vi "report_test_27_5_A86b2.vi"() -> ()   [LabVIEW 2021]
uses:
  <vilib>/Utility/NIReport.llb/NI_report.lvclass
  <vilib>/Platform/TimedLoop/XDataNode/timing_clust.ctl
  <vilib>/Platform/TimedLoop/XDataNode/nitl_modes.ctl
  <vilib>/Platform/TimedLoop/XDataNode/wakeup.ctl
  <vilib>/Utility/NIReport.llb/Report Type.ctl
  <extravilib>/ChannelInstances/Tag-dbl/Read With Abort.vi
  <extravilib>/ChannelInstances/Tag-a[.](dbl)/Write With Abort.vi
  <extravilib>/ChannelInstances/Tag-bool/Write With Abort.vi
  <extravilib>/ChannelInstances/Tag-bool/Read With Abort.vi
  <extravilib>/ChannelInstances/Tag-a[.](dbl)/Read With Abort.vi
  <extravilib>/ChannelInstances/Tag-dbl/Write With Abort.vi
  <extravilib>/ChannelInstances/Tag-dbl/Instantiate.vi
  <extravilib>/ChannelInstances/Tag-bool/Instantiate.vi
  <extravilib>/ChannelInstances/Tag-bool/EndpointRead.vi
  <vilib>/OPCUA/client/Multiple Read Float.vi
  <extravilib>/ChannelInstances/Tag-dbl/Endpoint.vi
  <extravilib>/ChannelInstances/Tag-a[.](dbl)/Instantiate.vi
  <extravilib>/ChannelInstances/Tag-bool/Endpoint.vi
  <extravilib>/ChannelInstances/Tag-a[.](dbl)/EndpointRead.vi
  <vilib>/Utility/file.llb/Write Delimited Spreadsheet (DBL).vi
  <vilib>/Utility/NIReport.llb/Append Numeric Table to Report (wrap).vi
  <extravilib>/ChannelInstances/Tag-dbl/EndpointRead.vi
  <extravilib>/ChannelInstances/Tag-a[.](dbl)/Endpoint.vi
  <vilib>/Platform/TimedLoop/XDataNode/XDataNode.xnode
  <vilib>/Platform/TimedLoop/XDataNode/XDNodeRunTimeDep.lvlib
  <extravilib>/ChannelInstances/Tag-bool.lvlib
  <vilib>/OPCUA/NI OPC UA Client.lvlib
  <vilib>/Utility/NIReport.llb/NI_ReportGenerationCore.lvlib
  <extravilib>/ChannelInstances/Tag-a[.](dbl).lvlib
  <extravilib>/ChannelInstances/Tag-dbl.lvlib
panel:
  in  "y 2":dbl=1.5
  out "x":dbl
  out "highqq":dbl(graph)
  out "Endpoint_Highqq":dbl
  out "velx":dbl(graph)
  out "x":dbl(graph)
  out "vx":dbl
  out "angle Y":dbl
  out "Endpoint_l":dbl[](array[numeric])
  out "Endpoint_lfull 2":dbl[][](array[numeric])
  in  "source file path":path=path "D:/Phuc/postopulsem2.m"
  out "appended array 2":dbl[](array[numeric])
  out "appended array":dbl[](array[numeric])
  out "data out 2":string
  in  "String":string="Flight_report"
  out "Gyro acc & vel":dbl[](array[numeric])
  out "Roll & Pitch":cluster{"[0]":dbl, "[1]":dbl}(graph)
  out "Cable length":T1(graph)
  out "Tilt sensor array":dbl[](array[numeric])
  out "Cable length Array":dbl[](array[numeric])
  in  "PAR_GpDec":dbl=120000.0
  in  "Set pos":bool caption="Blank Button"
  in  "Set cmd & actual pos":dbl[](array[numeric])=[0.0, 0.0, 0.0, 0.0, 0.0, 0.0, -2293.0, -3672.0]
  in  "CFG_GpSFEnable":u32(ring) items=["SF_Disable", "SF_Enable"]
  in  "Par":bool
  out "Ax = y?":bool
  in  "CFG_GpBldTime":u32
  in  "y":u32=1
  out "pCurIndex":u32
  out "pCurCmdFunc":u32
  out "pRemainCount":u32
  out "pFreeSpaceCount":u32
  out "Waveform Chart":T1(graph)
  out "Tensile force array":dbl[](array[numeric])
  out "Exel report":refnum<class "NI_report.lvclass">
  out "Roll":string
  out "Pitch":string
  out "Yaw":string="0"
  out "LinAcc X":string
  out "LinAcc Y":string
  out "LinAcc Z":string
  out "Cable velocity (m/s)":T1(graph)
  in  "Tab Control":enum32{"Page 1", "Page 2"}(tab)
  in  "Open Board":bool
  in  "Stop 2":bool
  out "Group State:":string
  in  "Servo On":bool
  in  "Adress":string="192.168.0.100"
  in  "Port 2":u16=3535
  in  "bytes to read 2":i32=32
  in  "Stop 3":bool
  in  "bytes to read":i32=72
  in  "Address":string="192.168.0.199"
  in  "Port":u16=8888
  in  "stop":bool
  in  "Clear report":bool
  in  "Save report":bool
  in  "Enable write":bool
  in  "Write to report":bool
  in  "Close Board":bool
  in  "trust any server (F)":bool=TRUE
  in  "Server endpoint URL":string="opc.tcp://127.0.0.1:49350"
  in  "NodeID 8":string="ns=2;s=S7.PLC4.loadcell7"
  in  "NodeID 7":string="ns=2;s=S7.PLC4.loadcell6"
  in  "NodeID 6":string="ns=2;s=S7.PLC3.loadcell5"
  in  "NodeID 5":string="ns=2;s=S7.PLC3.loadcell4"
  in  "NodeID 3":string="ns=2;s=S7.PLC2.loadcell2"
  in  "NodeID 4":string="ns=2;s=S7.PLC2.loadcell3"
  in  "NodeID 2":string="ns=2;s=S7.PLC1.loadcell1"
  in  "NodeID 1":string="ns=2;s=S7.PLC1.loadcell0"
  out "data out":string
  out "Measured tensile force (N)":T2(graph)
  out "Error Code:":u32 format="%x"
  out "Error Msg":string
  out "Error":bool
  in  "Reset Error":bool
  out "Instrument":string="If you want to exit program,Please press \"Exit Program\" button"
  out "DeviceNum List":u32[](array[numeric])
  out "Servo_Off":bool
  out "Servo_On":bool
  out "GPHandle":u64
  out "CFG_GpAxesInGroup":u32
  out "GroupClosed":bool
  out "GroupStopped":bool
  out "DirectAbsSuccess":bool
  out "DirectRelSuccess":bool
  in  "Movement Mode":enum32{"Absolute", "Relative"}(radio)=enum."Relative"
  out "GroupOpened":bool
  in  "Direct Ends":dbl[](array[numeric])=[10000.0, 10000.0, 10000.0, 10000.0, 10000.0, 10000.0, 10000.0, 10000.0]
  in  "Operate Axes":T3={"0-Axis"=TRUE, "1-Axis"=TRUE, "2-Axis"=TRUE, "3-Axis"=TRUE, "4-Axis"=TRUE, "5-Axis"=TRUE, "6-Axis"=TRUE, "7-Axis"=TRUE}
  out "CloseSuccess":bool
  in  "Device Type":u16(ring) items=["PCI-1285 (M0)"]
  out "Exit Program":bool
  out "DeviceOpened":bool
  out "AxisOpened":bool
  out "AxisHandle_Array":u64[](array[numeric])
  out "DevAxesCount":u32
  in  "Stop":bool
  in  "Direct":bool
  out "ResetCounter":bool
  in  "Reset Counter":bool
  out "Axis Position":T4
  out "DeviceHandle":u64
  # "MPU measurement"
  # "(deg)"
  # "(m/s^2)"
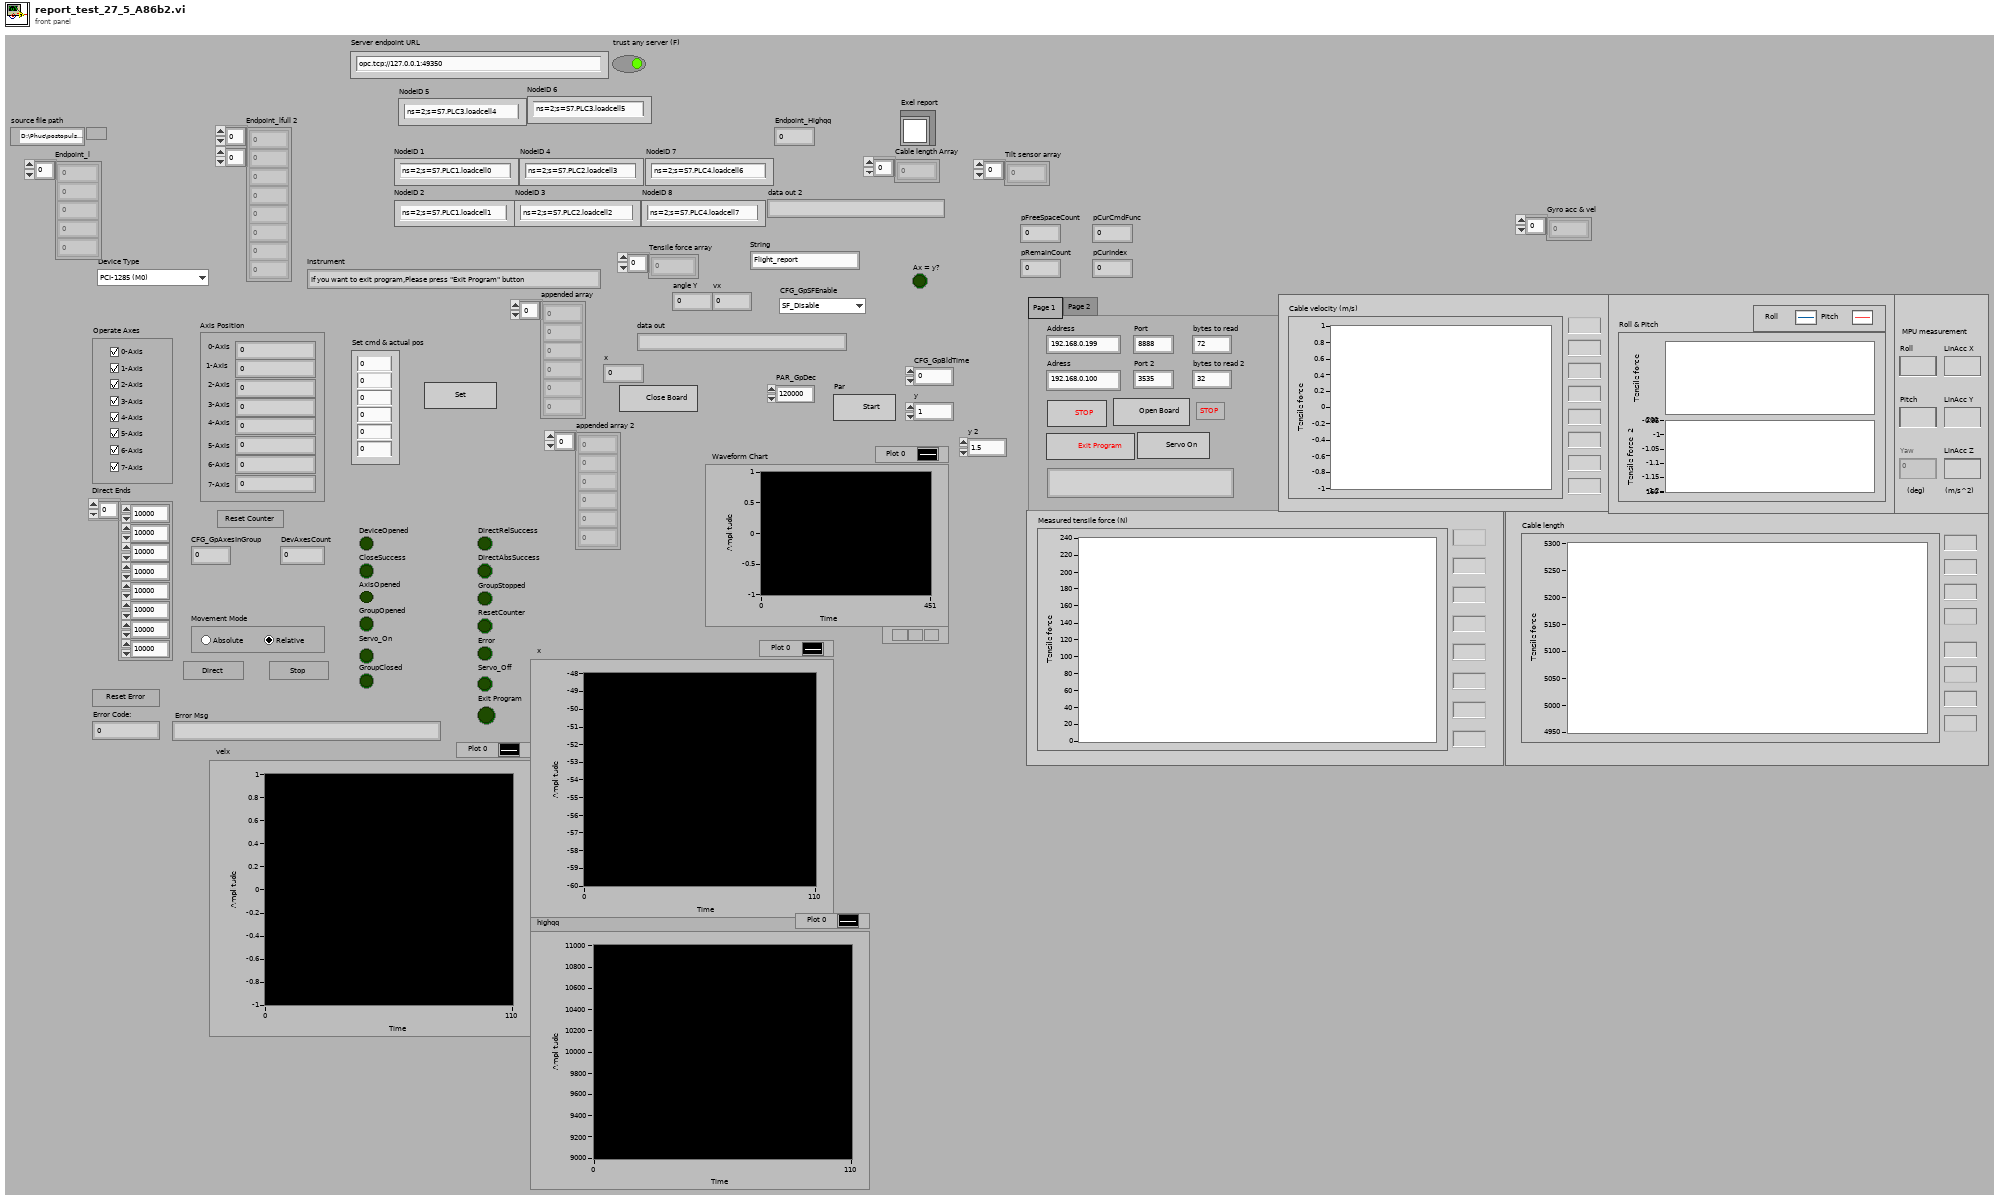
[diagram p1: front panel]
types:
  T1 = cluster{"[0]":dbl, "[1]":dbl, "[2]":dbl, "[3]":dbl, "[4]":dbl, "[5]":dbl, "[6]":dbl, "[7]":dbl}
  T2 = cluster{"[0]":sgl, "[1]":sgl, "[2]":sgl, "[3]":sgl, "[4]":sgl, "[5]":sgl, "[6]":sgl, "[7]":sgl}
  T3 = cluster{"0-Axis":bool, "1-Axis":bool, "2-Axis":bool, "3-Axis":bool, "4-Axis":bool, "5-Axis":bool, "6-Axis":bool, "7-Axis":bool}
  T4 = cluster{"0-Axis":dbl, "1-Axis":dbl, "2-Axis":dbl, "3-Axis":dbl, "4-Axis":dbl, "5-Axis":dbl, "6-Axis":dbl, "7-Axis":dbl}
  T5 = cluster{"message mode":enum16{"None", "Sign", "Sign and Encrypt"}, "security":enum16{"Basic256", "Basic128Rsa15"}}
  T6 = typedef "NI_ReportGenerationCore.lvlib/Report Type.ctl" = enum16{"HTML", "Word", "Excel"}
  T7 = enum16{"maximized", "minimized", "normal", "no change"}
  T8 = cluster{"DeviceNum":u32, "U*8 Array":cluster{"U*8 Array[0]":u8, "U*8 Array[1]":u8, "U*8 Array[2]":u8, "U*8 Array[3]":u8, "U*8 Array[4]":u8, "U*8 Array[5]":u8, "U*8 Array[6]":u8, "U*8 Array[7]":u8, "U*8 Array[8]":u8, "U*8 Array[9]":u8, "U*8 Array[10]":u8, "U*8 Array[11]":u8, "U*8 Array[12]":u8, "U*8 Array[13]":u8, "U*8 Array[14]":u8, "U*8 Array[15]":u8, "U*8 Array[16]":u8, "U*8 Array[17]":u8, "U*8 Array[18]":u8, "U*8 Array[19]":u8, "U*8 Array[20]":u8, "U*8 Array[21]":u8, "U*8 Array[22]":u8, "U*8 Array[23]":u8, "U*8 Array[24]":u8, "U*8 Array[25]":u8, "U*8 Array[26]":u8, "U*8 Array[27]":u8, "U*8 Array[28]":u8, "U*8 Array[29]":u8, "U*8 Array[30]":u8, "U*8 Array[31]":u8, "U*8 Array[32]":u8, "U*8 Array[33]":u8, "U*8 Array[34]":u8, "U*8 Array[35]":u8, "U*8 Array[36]":u8, "U*8 Array[37]":u8, "U*8 Array[38]":u8, "U*8 Array[39]":u8, "U*8 Array[40]":u8, "U*8 Array[41]":u8, "U*8 Array[42]":u8, "U*8 Array[43]":u8, "U*8 Array[44]":u8, "U*8 Array[45]":u8, "U*8 Array[46]":u8, "U*8 Array[47]":u8, "U*8 Array[48]":u8, "U*8 Array[49]":u8}, "NumOfSubDevice":i16}[]
  T9 = cluster{"U*8 Array[0]":u8, "U*8 Array[1]":u8, "U*8 Array[2]":u8, "U*8 Array[3]":u8, "U*8 Array[4]":u8, "U*8 Array[5]":u8, "U*8 Array[6]":u8, "U*8 Array[7]":u8, "U*8 Array[8]":u8, "U*8 Array[9]":u8, "U*8 Array[10]":u8, "U*8 Array[11]":u8, "U*8 Array[12]":u8, "U*8 Array[13]":u8, "U*8 Array[14]":u8, "U*8 Array[15]":u8, "U*8 Array[16]":u8, "U*8 Array[17]":u8, "U*8 Array[18]":u8, "U*8 Array[19]":u8, "U*8 Array[20]":u8, "U*8 Array[21]":u8, "U*8 Array[22]":u8, "U*8 Array[23]":u8, "U*8 Array[24]":u8, "U*8 Array[25]":u8, "U*8 Array[26]":u8, "U*8 Array[27]":u8, "U*8 Array[28]":u8, "U*8 Array[29]":u8, "U*8 Array[30]":u8, "U*8 Array[31]":u8, "U*8 Array[32]":u8, "U*8 Array[33]":u8, "U*8 Array[34]":u8, "U*8 Array[35]":u8, "U*8 Array[36]":u8, "U*8 Array[37]":u8, "U*8 Array[38]":u8, "U*8 Array[39]":u8, "U*8 Array[40]":u8, "U*8 Array[41]":u8, "U*8 Array[42]":u8, "U*8 Array[43]":u8, "U*8 Array[44]":u8, "U*8 Array[45]":u8, "U*8 Array[46]":u8, "U*8 Array[47]":u8, "U*8 Array[48]":u8, "U*8 Array[49]":u8}
  T10 = enum32{"Invalid", "Standard", "Closed", "Hidden", "Minimized", "Maximized"}
  T11 = typedef "XDNodeRunTimeDep.lvlib/timing_clust.ctl" = cluster{"Expected End [f-1]":u64, "Actual End [f-1]":u64, "Finished Late? [f-1]":bool, "Expected End [i-1]":u64, "Actual End [i-1]":u64, "Finished Late? [i-1]":bool, "Expected Start [i]":u64, "Actual Start [i]":u64, "Expected Start [f]":u64, "Actual Start [f]":u64, "Source Name":string, "Structure Name":string, "Period":i64, "Deadline":i64, "Offset":i64, "Start":i64, "Priority":i32, "Timeout":i32, "Mode":T12, "Wakeup Reason":T13, "Error":errorcluster, "Source Type":string, "Secondary Source Type":string, "Global End Time":u64, "Global Start Time":u64, "Frame Duration":u64, "Iteration Duration":u64, "Assigned CPU":i32, "I/O Scan Engine Mode":u32}
  T12 = typedef "XDNodeRunTimeDep.lvlib/nitl_modes.ctl" = enum32{"No Change", "Process missed periods, maintain original phase", "Discard missed periods, maintain original phase", "Process missed periods, ignore original phase", "Discard missed periods, ignore original phase"}
  T13 = typedef "XDNodeRunTimeDep.lvlib/wakeup.ctl" = enum32{"Normal", "Aborted", "Asynchronous wakeup", "Timing source error", "Timed loop error", "Timeout"}
  T14 = typedef "OPC UA Client Refnum.ctl" = refnum<k21>
  T15 = typedef "Tag-dbl.lvlib/))Channel.ctl" = refnum<queue>
  T16 = cluster{"Endpoint_lfull":dbl[][], "Endpoint_l":dbl[], "Endpoint_Highqq":dbl}
  T17 = typedef "Tag-a[.](dbl).lvlib/))Channel.ctl" = refnum<queue>
  T18 = typedef "Tag-bool.lvlib/))Channel.ctl" = refnum<queue>
  T19 = cluster{"position (excel)":cluster{"row":i32, "column":i32}, "name (excel)":string, "bookmark (word)":string}
  T20 = typedef "NodeId.ctl" = string
  T21 = typedef "OPC UA StatusCode.ctl" = u32
  T22 = cluster{"node ID":T20, "value ":sgl, "timestamp":timestamp, "status":T21}[]
  T23 = cluster{"node ID":T20, "value ":sgl, "timestamp":timestamp, "status":T21}
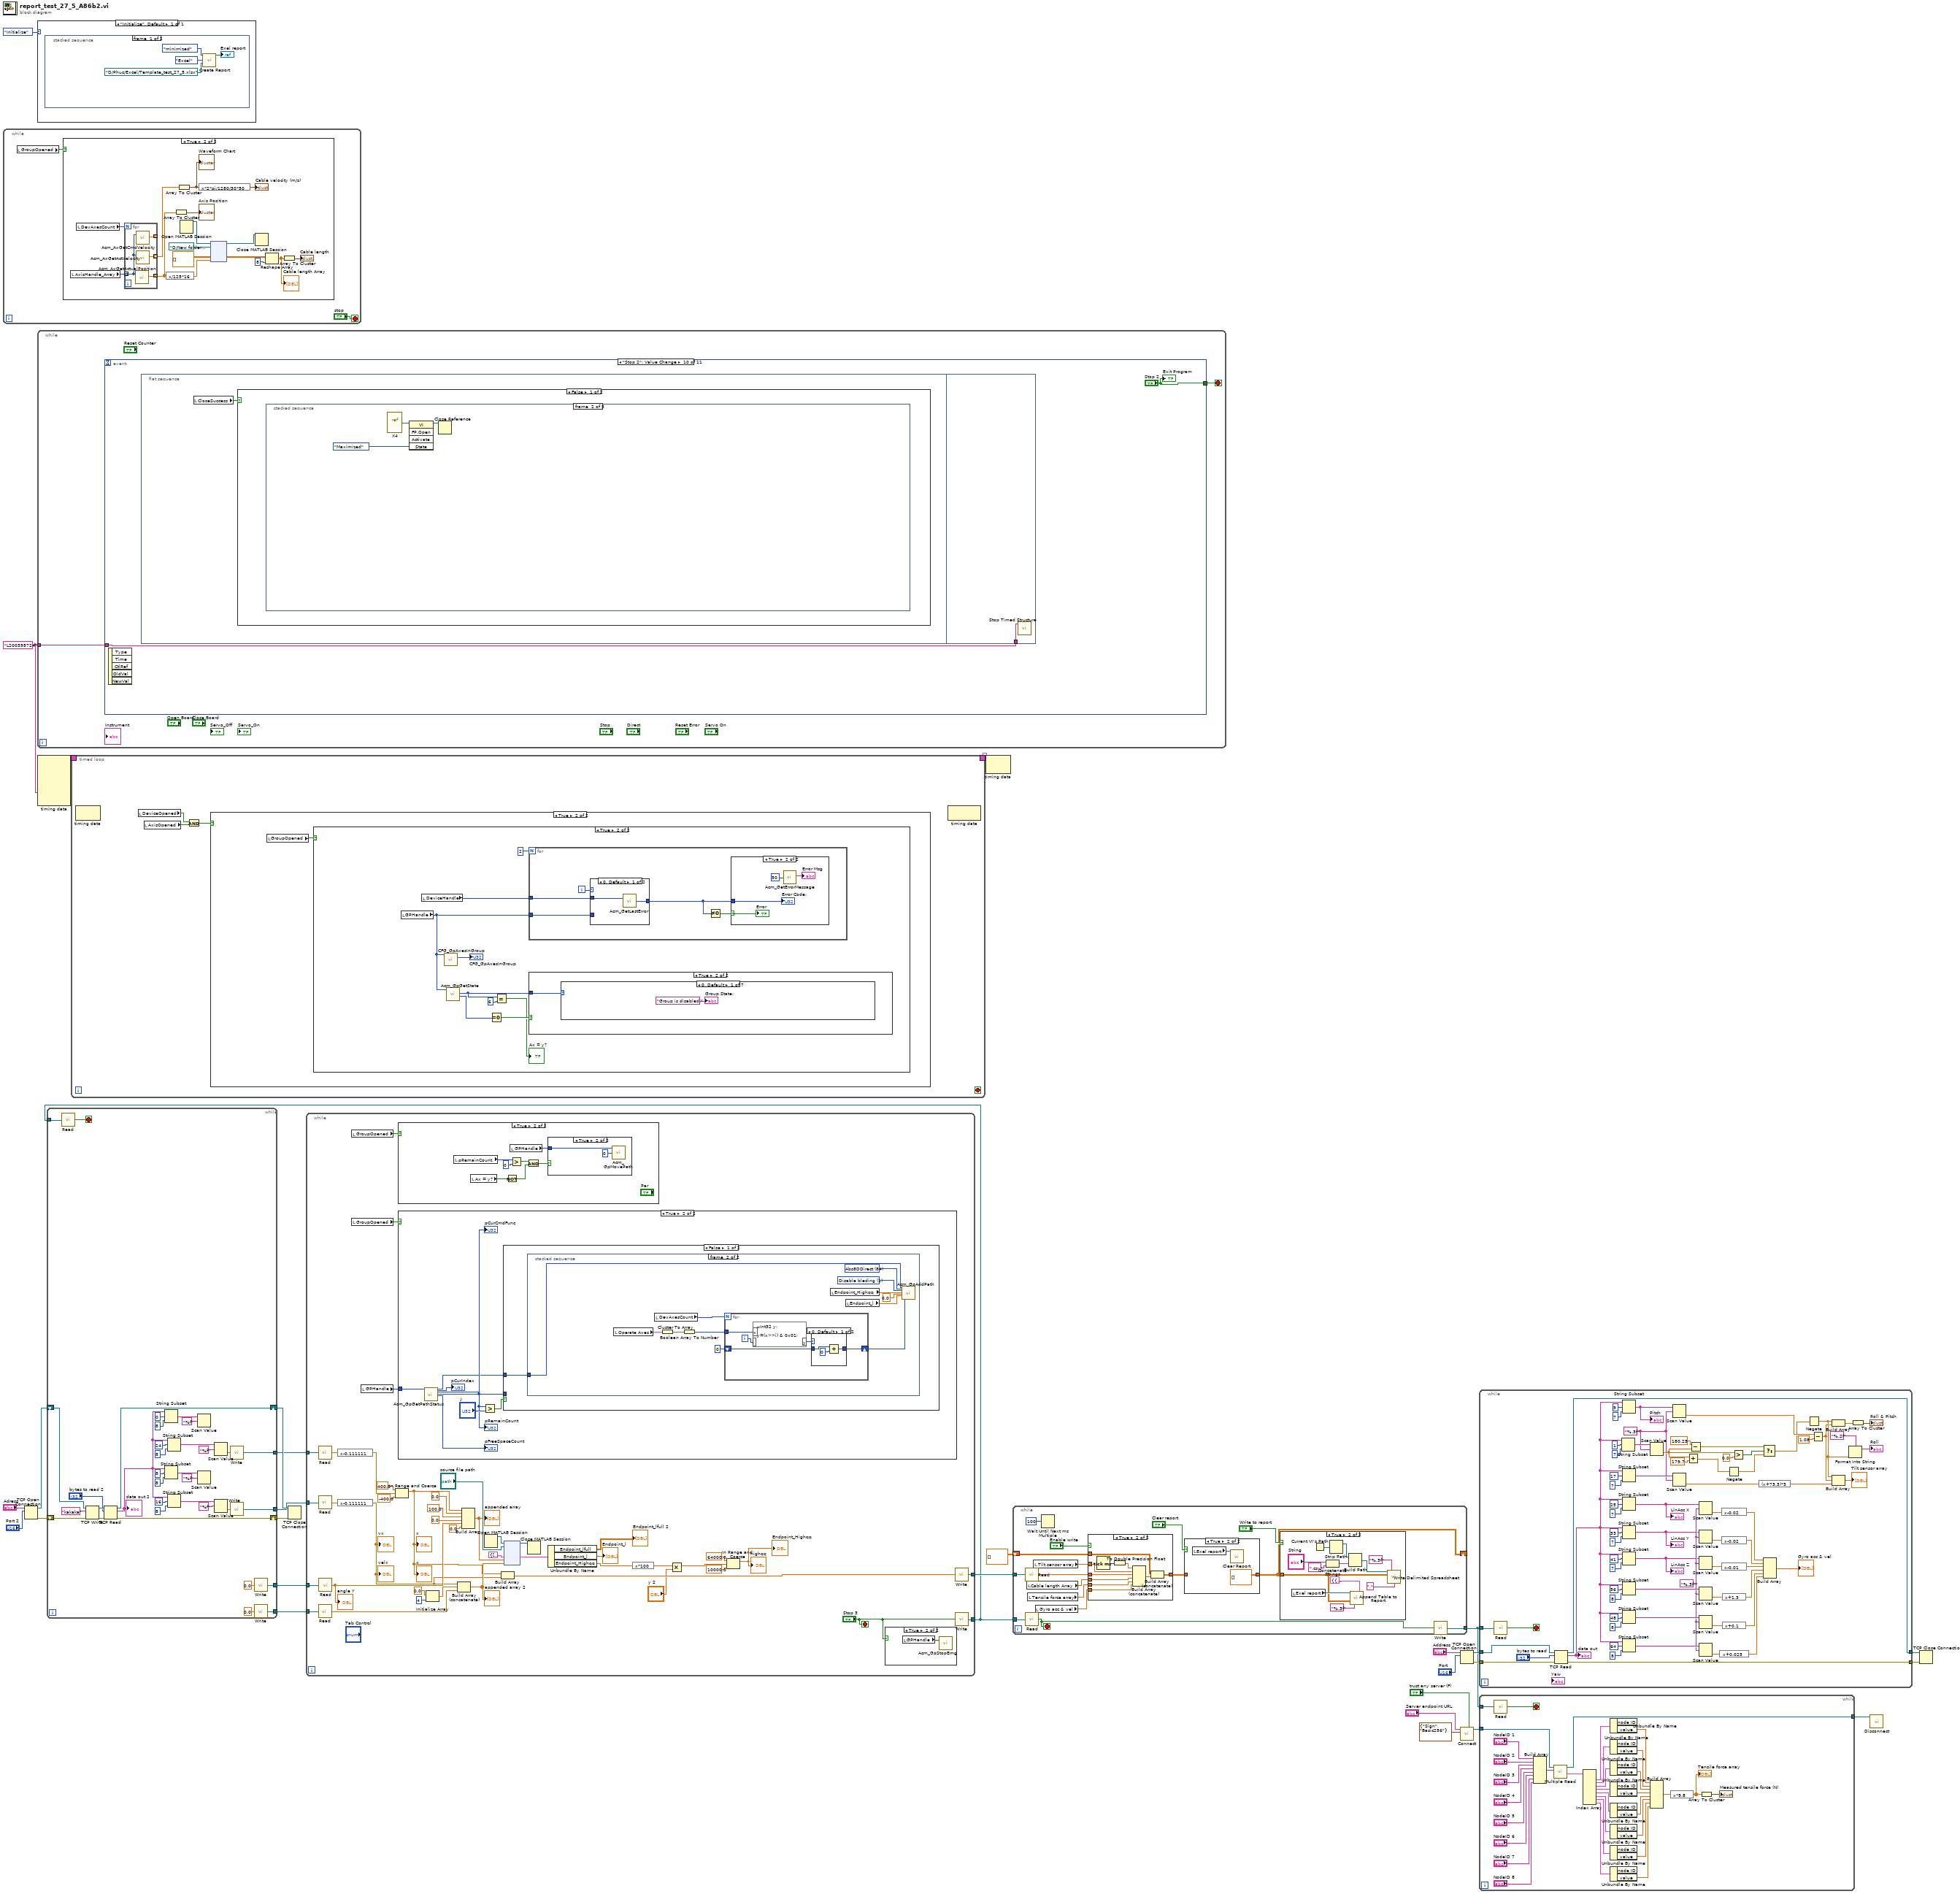
[diagram p0: block diagram]
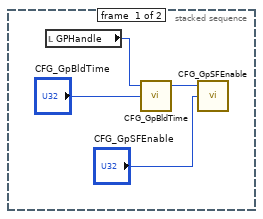
[diagram p9: hidden frame]
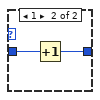
[diagram p10: hidden frame]
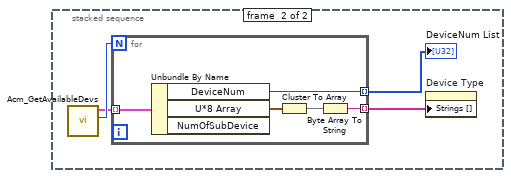
[diagram p13: hidden frame]
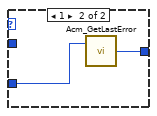
[diagram p17: hidden frame]
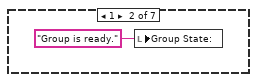
[diagram p19: hidden frame]
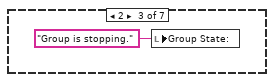
[diagram p20: hidden frame]
diagram:
  w27 = "L200395724" ("结构名称")
  n1 = while {
    stop <- "stop" stop-if-true
    n2 = local read "GroupOpened"() -> (w31:bool)
    n3 = case shown="True" w31 {
      frame False {
      }
      frame True {
        n4 = local read "AxisHandle_Array"() -> (w47:u64[])
        n5 = local read "DevAxesCount"() -> (w44:u32)
        n6 = for {
          N: w44 -> [_]
          tunnel: [w50] -> w41 mode=indexing
          tunnel: [w51] -> w46 mode=indexing
          tunnel: [w49] -> _ mode=indexing
          tunnel: w47 -> [w48] mode=indexing
          n7 = call <userlib>:"Acm_AxGetActualPosition.vi"("AxisHandle"=w48) -> ("Position"=w50:dbl)  [unwired: 1 in, 3 out]
          n8 = call <userlib>:"Acm_AxGetCmdVelocity.vi"("AxisHandle"=w48) -> ("Velocity"=w49:dbl)  [unwired: 1 in, 3 out]
          n9 = call <userlib>:"Acm_AxGetActVelocity.vi"("AxisHandle"=w48) -> ("Velocity"=w51:dbl)  [unwired: 1 in, 3 out]
        }
        n10 = expression code="x/125*16"(w41) -> (w40:dbl[])
        n11 = Array To Cluster(array=w41) -> (cluster=→"Axis Position":T1)
        n12 = Array To Cluster(array=w46) -> (cluster=w42:T1)
        "Waveform Chart" <- w42
        n13 = Open MATLAB Session() -> (8:w36:refnum<k37>)  [unwired: 2 in, 1 out]
        n14 = expression code="x*2*pi/1280/30*50"(w42) -> (→"Cable velocity (m/s)":T1)
        n15 = node(w36, path "D:/New folder/Cap_length.m" ("source file path"), dbl[][] [], w40) -> (w39:refnum<k37>, w34:dbl[][])  [unwired: 3 in, 3 out]
        n16 = Close MATLAB Session(0:w39) -> ()  [unwired: 1 in, 1 out]
        n17 = Reshape Array(w34, 8 ("dimension size")) -> (w32:dbl[])
        "Cable length Array" <- w32
        n18 = Array To Cluster(array=w32) -> (cluster=→"Cable length":T1)
      }
    }
  }
  n19 = TCP Open Connection(address="Adress", remote port or service name="Port 2") -> (connection ID=w21:refnum<k5>, error out=w22:errorcluster)  [unwired: 3 in]
  n20 = case shown="\"Initialize\", Default" enum16{"Initialize"}."Initialize" ("Enum") {
    frame "Initialize", Default {
      n21 = stacked-sequence {
        frame #0 {
          n22 = call <vilib>:"Create Report.vi"("window state (normal)"=T7."minimized", "report type"=Report_Type."Excel", "template (empty)"=path "D:/Phuc/Excel/Template_test_27_5.xlsx") -> ("report out"=→"Exel report":refnum<class "NI_report.lvclass">)  [unwired: 11 in, 1 out]
        }
        frame #1 {
          n23 = call <userlib>:"Acm_GetAvailableDevs.vi"() -> ("DeviceList"=w58:T8, "OutEntries"=w59:u32)  [unwired: 1 in, 4 out]
          n24 = for {
            N: w59 -> [_]
            tunnel: w58 -> [w64] mode=indexing
            tunnel: [w61] -> w57 mode=indexing
            tunnel: [w60] -> w56 mode=indexing
            n25 = Unbundle By Name(w64) -> ("DeviceNum"=w61:u32, "U*8 Array"=w63:T9)  [unwired: 1 out]
            n26 = Cluster To Array(cluster=w63) -> (array=w62:u8[])
            n27 = Byte Array To String(unsigned byte array=w62) -> (string=w60:string)
          }
          "DeviceNum List" <- w57
          n28 = property on="Device Type" class="Ring (strict)"("Strings []"=w56) -> ()  [unwired: 2 in, 2 out]
        }
      }
    }
  }
  n29 = while {
    tunnel: w27 -> [w66]
    stop <- w65 stop-if-true
    n30 = event shown="[9] \"Stop 2\": Value Change" {
      selector: _ -> [_ _ _ _ _ _ _ _ _ _ _]
      dyn-events: _ -> [_ _ _ _ _ _ _ _ _ _ _]
      timeout: _ -> [_ _ _ _ _ _ _ _ _ _ _]
      tunnel: w66 -> [_ _ _ _ _ _ _ _ _ w257 _]
      tunnel: [_ _ _ _ _ _ _ _ _ "Stop 2" _] -> w65
      event "Open Board": Mouse Up {
        n31 = event-data() -> ()  [unwired: 8 out]
        n32 = local read "DeviceNum List"() -> (w71:u32[])
        n33 = local read "Device Type"() -> (w70:u16)
        n34 = Index Array(array=w71, index=w70) -> (element=w69:u32)
        n35 = call <userlib>:"Acm_DevOpen.vi"("DeviceNumber"=w69) -> ("ReturnValue"=w67:u32, "DeviceHandle"=→"DeviceHandle":u64)  [unwired: 1 in, 1 out]
        n36 = Equal?(x=w67, y=u32 0) -> (x = y?=w68:bool)
        "DeviceOpened" <- w68
        n37 = stacked-sequence {
          tunnel: w68 -> [w79 _ _]
          frame #0 {
            n38 = case shown="True" w79 {
              frame False {
              }
              frame True {
                n39 = local read "DeviceHandle"() -> (w81:u64)
                n40 = call <userlib>:"FT_DevAxesCount.vi"("Handle"=w81) -> ("DevAxesCount"=w82:u32)  [unwired: 1 in, 13 out]
                "DevAxesCount" <- w82
                n41 = for {
                  N: w82 -> [_]
                  tunnel: w81 -> [w87]
                  tunnel: [w83] -> w80 mode=indexing
                  i -> [w86]
                  n42 = call <userlib>:"Acm_AxOpen.vi"("PhyAxis"=w86, "DeviceHandle"=w87) -> ("ReturnValue"=w85:u32, "AxisHandle"=w83:u64)  [unwired: 1 in, 2 out]
                  n43 = Equal To 0?(x=w85) -> (x = 0?=→"AxisOpened":bool)
                }
                "AxisHandle_Array" <- w80
              }
            }
          }
          frame #1 {
            n44 = local read "AxisOpened"() -> (w88:bool)
            n45 = case shown="True" w88 {
              frame False {
              }
              frame True {
                n46 = Cluster To Array(cluster="Operate Axes") -> (array=w92:bool[])
                n47 = local read "DevAxesCount"() -> (w89:u32)
                n48 = Boolean Array To Number(Boolean array=w92) -> (number=w90:u32)
                n49 = for {
                  N: w89 -> [_]
                  tunnel: w90 -> [w95]
                  i -> [w93]
                  n50 = formula code="uInt32 y;\n\ny=(x>>i) & 0x01;"("x"=w95, "i"=w93) -> ("y"=w94:u32)
                  n51 = case shown="1" w94 {
                    tunnel: w93 -> [_ w102]
                    frame 0, Default {
                    }
                    frame 1 {
                      n52 = local read "AxisHandle_Array"() -> (w103:u64[])
                      n53 = local read "GPHandle"() -> (w97:u64)
                      n54 = Index Array(array=w103, index=w102) -> (element=w101:u64)
                      n55 = call <userlib>:"Acm_GpAddAxis.vi"("AxHandle"=w101, "GPHandle"=w97) -> ("ReturnValue"=w99:u32, "GPHandle"=→"GPHandle":u64)  [unwired: 1 in, 1 out]
                      n56 = Equal To 0?(x=w99) -> (x = 0?=w100:bool)
                      "GroupOpened" <- w100
                      n57 = Not(x=w100) -> (.not. x?=w96:bool)
                      n58 = case shown="True" w96 {
                        tunnel: w99 -> [_ w109]
                        frame False {
                        }
                        frame True {
                          n59 = local read "GPHandle"() -> (w105:u64)
                          n60 = Not Equal To 0?(x=w105) -> (x != 0?=w104:bool)
                          n61 = case shown="True" w104 {
                            frame False {
                            }
                            frame True {
                              n62 = local write "GroupOpened"(TRUE) -> ()
                            }
                          }
                          n63 = Number To Hexadecimal String(2:w109) -> (0:w107:string)  [unwired: 1 out]
                          n64 = Concatenate Strings("Group Add Axis Failed With Error Code:0x", w107) -> (w106:string)
                          n65 = One Button Dialog(message=w106) -> ()  [unwired: 2 out]
                        }
                      }
                      n66 = local write "GroupClosed"(w96) -> ()
                    }
                  }
                }
              }
            }
          }
          frame #2 {
            n67 = local read "GPHandle"() -> (w112:u64)
            n68 = call <userlib>:"PAR_GpDec.vi"("PAR_GpDec"="PAR_GpDec", "Handle"=w112) -> ()  [unwired: 1 in, 3 out]
            n69 = call <userlib>:"PAR_GpAcc.vi"("PAR_GpAcc"="PAR_GpDec", "Handle"=w112) -> ()  [unwired: 1 in, 3 out]
          }
        }
        n70 = Not(x=w68) -> (.not. x?=w74:bool)
        n71 = case shown="True" w74 {
          tunnel: w67 -> [_ w75]
          frame False {
          }
          frame True {
            n72 = Number To Hexadecimal String(2:w75) -> (0:w77:string)  [unwired: 1 out]
            n73 = Concatenate Strings("Open Board Failed With Error Code:0x", w77) -> (w76:string)
            n74 = One Button Dialog(message=w76) -> ()  [unwired: 2 out]
          }
        }
        n75 = local write "CloseSuccess"(w74) -> ()
      }
      event "Device Type": Value Change {
        n76 = event-data() -> ()  [unwired: 6 out]
        n77 = local write "Device Type"("Device Type") -> ()
      }
      event "Servo On": Value Change {
        n78 = event-data() -> ()  [unwired: 6 out]
        n79 = local read "DevAxesCount"() -> (w114:u32)
        n80 = for {
          N: w114 -> [_]
          i -> [w123]
          n81 = local read "Servo On"() -> (w122:bool)
          n82 = case shown="False" w122 {
            tunnel: [u32 0 u32 1] -> w120
            frame False {
            }
            frame True {
            }
          }
          n83 = local read "AxisHandle_Array"() -> (w124:u64[])
          n84 = Index Array(array=w124, index=w123) -> (element=w121:u64)
          n85 = call <userlib>:"Acm_AxSetSvOn.vi"("OnOff"=w120, "AxisHandle"=w121) -> ("ReturnValue"=w115:u32)  [unwired: 1 in, 2 out]
          n86 = Not Equal To 0?(x=w115) -> (x != 0?=w119:bool)
          n87 = case shown="True" w119 {
            tunnel: w115 -> [_ w129]
            frame False {
            }
            frame True {
              w132 = "Servo On/Off Failed With Error Code:0x"  # Servo On/Off Failed With Error Code:0x
              n88 = Number To Hexadecimal String(2:w129) -> (0:w131:string)  [unwired: 1 out]
              n89 = Concatenate Strings(w132, w131) -> (w130:string)
              n90 = One Button Dialog(message=w130) -> ()  [unwired: 2 out]
            }
          }
          n91 = Not(x=w119) -> (.not. x?=w118:bool)
          n92 = local read "Servo On"() -> (w117:bool)
          n93 = And(x=w117, y=w118) -> (x .and. y?=w116:bool)
          n94 = case shown="True" w116 {
            frame False {
              n95 = local write "Servo_Off"(TRUE ("Servo_Off")) -> ()
              n96 = local write "Servo_On"(FALSE ("Servo_On")) -> ()
            }
            frame True {
              n97 = local write "Servo_On"(TRUE ("Servo_On")) -> ()
              n98 = local write "Servo_Off"(FALSE ("Servo_Off")) -> ()
            }
          }
        }
      }
      event "Operate Axes": Value Change {
        n99 = event-data() -> ()  [unwired: 6 out]
        n100 = local read "Operate Axes"() -> (w139:T3)
        n101 = local read "CFG_GpAxesInGroup"() -> (w135:u32)
        n102 = Cluster To Array(cluster=w139) -> (array=w137:bool[])
        n103 = local read "DevAxesCount"() -> (w138:u32)
        n104 = Boolean Array To Number(Boolean array=w137) -> (number=w136:u32)
        n105 = for {
          N: w138 -> [_]
          tunnel: w136 -> [w144]
          tunnel: w135 -> [w143]
          i -> [w140]
          n106 = formula code="uInt32 b,c,y1,y2;\n\nb=(x>>i) & 0x01;\nc=(a>>i) & 0x01;\nif((b==1)&&(c==0))\n{\ny1=1;\n}\nelse if((b==0)&(c==1))\n{\n y2=1;\n}"("x"=w144, "i"=w140, "a"=w143) -> ("y1"=w142:u32, "y2"=w141:u32)
          n107 = case shown="1" w141 {
            tunnel: w140 -> [_ w146]
            frame 0, Default {
            }
            frame 1 {
              n108 = local read "AxisHandle_Array"() -> (w147:u64[])
              n109 = local read "GPHandle"() -> (w148:u64)
              n110 = Index Array(array=w147, index=w146) -> (element=w145:u64)
              n111 = call <userlib>:"Acm_GpRemAxis.vi"("AxHandle"=w145, "GpHandle"=w148) -> ()  [unwired: 1 in, 4 out]
            }
          }
          n112 = case shown="1" w142 {
            tunnel: w140 -> [_ w155]
            frame 0, Default {
            }
            frame 1 {
              n113 = local read "AxisHandle_Array"() -> (w156:u64[])
              n114 = local read "GPHandle"() -> (w149:u64)
              n115 = Index Array(array=w156, index=w155) -> (element=w154:u64)
              n116 = call <userlib>:"Acm_GpAddAxis.vi"("AxHandle"=w154, "GPHandle"=w149) -> ("ReturnValue"=w152:u32, "GPHandle"=w150:u64)  [unwired: 1 in, 1 out]
              n117 = local write "GPHandle"(w150) -> ()
              n118 = Equal?(x=w152, y=0) -> (x = y?=w151:bool)
              n119 = local write "GroupOpened"(w151) -> ()
            }
          }
        }
      }
      event "Direct": Mouse Up {
        n120 = event-data() -> ()  [unwired: 8 out]
        n121 = local read "GroupOpened"() -> (w157:bool)
        n122 = case shown="True" w157 {
          frame False {
          }
          frame True {
            n123 = local read "Operate Axes"() -> (w164:T3)
            n124 = Cluster To Array(cluster=w164) -> (array=w163:bool[])
            n125 = local read "DevAxesCount"() -> (w158:u32)
            n126 = Boolean Array To Number(Boolean array=w163) -> (number=w162:u32)
            n127 = for {
              N: w158 -> [_]
              tunnel: w162 -> [w189]
              shift-right: [w185] -> w160
              shift-left: u32 0 -> [w186]
              i -> [w187]
              n128 = formula code="uInt32 y;\n\ny=(x>>i) & 0x01;"("x"=w189, "i"=w187) -> ("y"=w188:u32)
              n129 = case shown="0, Default" w188 {
                tunnel: w186 -> [w191 w194]
                tunnel: [w190 w193] -> w185
                frame 0, Default {
                  n130 = Add(x=w191, y=u32 0) -> (x+y=w190:u32)
                }
                frame 1 {
                  n131 = Increment(x=w194) -> (x+1=w193:u32)
                }
              }
            }
            n132 = case shown="\"Absolute\", Default" "Movement Mode" {
              tunnel: w160 -> [w165 w176]
              frame "Absolute", Default {
                n133 = local read "Direct Ends"() -> (w166:dbl[])
                n134 = local read "GPHandle"() -> (w170:u64)
                n135 = call <userlib>:"Acm_GpMoveDirectAbs.vi"("pArrayElements"=w165, "PositionArray"=w166, "GpHandle"=w170) -> ("ReturnValue"=w167:u32)  [unwired: 1 in, 2 out]
                n136 = Equal To 0?(x=w167) -> (x = 0?=w169:bool)
                "DirectAbsSuccess" <- w169
                n137 = Not(x=w169) -> (.not. x?=w168:bool)
                n138 = case shown="True" w168 {
                  tunnel: w167 -> [_ w174]
                  frame False {
                  }
                  frame True {
                    n139 = Number To Hexadecimal String(2:w174) -> (0:w172:string)  [unwired: 1 out]
                    n140 = Concatenate Strings("Direct Absolutely Failed With Error Code:0x", w172) -> (w171:string)
                    n141 = One Button Dialog(message=w171) -> ()  [unwired: 2 out]
                  }
                }
              }
              frame "Relative" {
                n142 = local read "GPHandle"() -> (w180:u64)
                n143 = call <userlib>:"Acm_GpMoveDirectRel.vi"("pArrayElements"=w176, "DistanceArray"="Direct Ends", "GpHandle"=w180) -> ("ReturnValue"=w177:u32)  [unwired: 1 in, 2 out]
                n144 = Equal To 0?(x=w177) -> (x = 0?=w179:bool)
                "DirectRelSuccess" <- w179
                n145 = Not(x=w179) -> (.not. x?=w178:bool)
                n146 = case shown="True" w178 {
                  tunnel: w177 -> [_ w184]
                  frame False {
                  }
                  frame True {
                    n147 = Number To Hexadecimal String(2:w184) -> (0:w182:string)  [unwired: 1 out]
                    n148 = Concatenate Strings("Direct Relatively failed with Error Code:0x", w182) -> (w181:string)
                    n149 = One Button Dialog(message=w181) -> ()  [unwired: 2 out]
                  }
                }
              }
            }
          }
        }
      }
      event "Stop": Mouse Up {
        n150 = event-data() -> ()  [unwired: 8 out]
        n151 = local read "GroupOpened"() -> (w195:bool)
        n152 = case shown="True" w195 {
          frame False {
          }
          frame True {
            n153 = local read "GPHandle"() -> (w199:u64)
            n154 = call <userlib>:"Acm_GpStopEmg.vi"("GpHandle"=w199) -> ("ReturnValue"=w196:u32)  [unwired: 1 in, 2 out]
            n155 = Equal To 0?(x=w196) -> (x = 0?=w198:bool)
            "GroupStopped" <- w198
            n156 = Not(x=w198) -> (.not. x?=w197:bool)
            n157 = case shown="True" w197 {
              tunnel: w196 -> [_ w203]
              frame False {
              }
              frame True {
                n158 = Number To Hexadecimal String(2:w203) -> (0:w201:string)  [unwired: 1 out]
                n159 = Concatenate Strings("Group Stop Failed With Error Code:0x", w201) -> (w200:string)
                n160 = One Button Dialog(message=w200) -> ()  [unwired: 2 out]
              }
            }
          }
        }
      }
      event "Reset Counter": Mouse Up {
        n161 = event-data() -> ()  [unwired: 8 out]
        n162 = local read "AxisOpened"() -> (w204:bool)
        n163 = case shown="True" w204 {
          frame False {
          }
          frame True {
            n164 = local read "DevAxesCount"() -> (w205:u32)
            n165 = for {
              N: w205 -> [_]
              i -> [w210]
              w207 = 0.0 ("Position")
              n166 = local read "AxisHandle_Array"() -> (w211:u64[])
              n167 = Index Array(array=w211, index=w210) -> (element=w206:u64)
              n168 = call <userlib>:"Acm_AxSetActualPosition.vi"("Position"=w207, "AxisHandle"=w206) -> ()  [unwired: 1 in, 3 out]
              n169 = call <userlib>:"Acm_AxSetCmdPosition.vi"("Position"=w207, "AxisHandle"=w206) -> ("ReturnValue"=w209:u32)  [unwired: 1 in, 2 out]
              n170 = Equal To 0?(x=w209) -> (x = 0?=→"ResetCounter":bool)
            }
          }
        }
      }
      event "Reset Error": Mouse Up {
        n171 = event-data() -> ()  [unwired: 9 out]
        n172 = local read "AxisOpened"() -> (w213:bool)
        n173 = local read "GroupOpened"() -> (w212:bool)
        n174 = case shown="True" w213 {
          frame False {
          }
          frame True {
            n175 = local read "Operate Axes"() -> (w215:T3)
            n176 = Cluster To Array(cluster=w215) -> (array=w216:bool[])
            n177 = local read "AxisHandle_Array"() -> (w219:u64[])
            n178 = Boolean Array To Number(Boolean array=w216) -> (number=w217:u32)
            n179 = Index Array(array=w219, index=w217) -> (element=w218:u64)
            n180 = call <userlib>:"Acm_AxResetError.vi"("AxisHandle"=w218) -> ()  [unwired: 1 in, 3 out]
          }
        }
        n181 = case shown="True" w212 {
          frame False {
          }
          frame True {
            n182 = local read "GPHandle"() -> (w214:u64)
            n183 = call <userlib>:"Acm_GpResetError.vi"("GpHandle"=w214) -> ()  [unwired: 1 in, 3 out]
          }
        }
      }
      event "Close Board": Mouse Up {
        n184 = event-data() -> ()  [unwired: 8 out]
        n185 = local read "DeviceOpened"() -> (w220:bool)
        n186 = case shown="True" w220 {
          frame False {
          }
          frame True {
            n187 = stacked-sequence {
              frame #0 {
                n188 = local read "GroupOpened"() -> (w221:bool)
                n189 = case shown="True" w221 {
                  frame False {
                  }
                  frame True {
                    n190 = local read "GPHandle"() -> (w225:u64)
                    n191 = call <userlib>:"Acm_GpClose.vi"("pGpHandle"=w225) -> ("ReturnValue"=w223:u32)  [unwired: 1 in, 1 out]
                    n192 = Equal To 0?(x=w223) -> (x = 0?=w222:bool)
                    "GroupClosed" <- w222
                    n193 = case shown="True" w222 {
                      selector: w222 -> [_ w229]
                      frame False {
                      }
                      frame True {
                        n194 = Not(x=w229) -> (.not. x?=w228:bool)
                        n195 = local write "GPHandle"(u32 0 ("GPHandle")) -> ()
                        n196 = local write "CFG_GpAxesInGroup"(u32 0 ("CFG_GpAxesInGroup")) -> ()
                        n197 = local write "GroupOpened"(w228) -> ()
                        n198 = local write "DirectRelSuccess"(w228) -> ()
                        n199 = local write "GroupStopped"(w228) -> ()
                        n200 = local write "DirectAbsSuccess"(w228) -> ()
                      }
                    }
                    n201 = Not(x=w222) -> (.not. x?=w224:bool)
                    n202 = case shown="True" w224 {
                      tunnel: w223 -> [_ w233]
                      frame False {
                      }
                      frame True {
                        n203 = Number To Hexadecimal String(2:w233) -> (0:w231:string)  [unwired: 1 out]
                        n204 = Concatenate Strings("Group Close failed with Error Code:0x", w231) -> (w230:string)
                        n205 = One Button Dialog(message=w230) -> ()  [unwired: 2 out]
                      }
                    }
                  }
                }
              }
              frame #1 {
                n206 = local read "DevAxesCount"() -> (w234:u32)
                n207 = for {
                  N: w234 -> [_]
                  i -> [w239]
                  n208 = local read "AxisHandle_Array"() -> (w240:u64[])
                  n209 = Index Array(array=w240, index=w239) -> (element=w238:u64)
                  n210 = call <userlib>:"Acm_AxClose.vi"("AxisHandle"=w238) -> ("ReturnValue"=w237:u32)  [unwired: 1 in, 1 out]
                  n211 = Equal To 0?(x=w237) -> (x = 0?=w236:bool)
                  n212 = Not(x=w236) -> (.not. x?=w235:bool)
                  n213 = local write "AxisOpened"(w235) -> ()
                }
              }
              frame #2 {
                n214 = local read "DeviceHandle"() -> (w244:u64)
                n215 = call <userlib>:"Acm_DevClose.vi"("DeviceHandle"=w244) -> ("ReturnValue"=w243:u32)  [unwired: 1 in, 3 out]
                n216 = Equal To 0?(x=w243) -> (x = 0?=w242:bool)
                "CloseSuccess" <- w242
                n217 = case shown="True" w242 {
                  tunnel: w242 -> [_ w251]
                  frame False {
                  }
                  frame True {
                    n218 = local write "GPHandle"(u32 0 ("GPHandle")) -> ()
                    n219 = local write "DeviceHandle"(u32 0 ("DeviceHandle")) -> ()
                    n220 = local write "DevAxesCount"(u32 0 ("DevAxesCount")) -> ()
                    n221 = Not(x=w251) -> (.not. x?=w250:bool)
                    n222 = local write "AxisOpened"(w250) -> ()
                    n223 = local write "DeviceOpened"(w250) -> ()
                    n224 = local write "ResetCounter"(w250) -> ()
                    n225 = local read "DevAxesCount"() -> (w254:u32)
                    n226 = Initialize Array(u32 0 ("元素"), w254) -> (w253:u32[])
                    n227 = local write "AxisHandle_Array"(w253) -> ()
                  }
                }
                n228 = Not(x=w242) -> (.not. x?=w241:bool)
                n229 = case shown="True" w241 {
                  tunnel: w243 -> [_ w245]
                  frame False {
                  }
                  frame True {
                    n230 = Number To Hexadecimal String(2:w245) -> (0:w247:string)  [unwired: 1 out]
                    n231 = Concatenate Strings("Close Board Failed With Error Code:0x", w247) -> (w246:string)
                    n232 = One Button Dialog(message=w246) -> ()  [unwired: 2 out]
                  }
                }
              }
            }
          }
        }
      }
      event "Stop 2": Value Change {
        n233 = event-data() -> ()  [unwired: 6 out]
        n234 = flat-sequence {
          tunnel: w257 -> [w297]
          frame #0 {
            n235 = local read "CloseSuccess"() -> (w259:bool)
            n236 = case shown="False" w259 {
              frame False {
                n237 = stacked-sequence {
                  frame #0 {
                    n238 = case shown="True" "Save report" {
                      frame False {
                      }
                      frame True {
                        n239 = local read "Exel report"() -> (w262:refnum<class "NI_report.lvclass">)
                        n240 = call-dynamic "Save Report to File.vi"("report in"=w262, "report file path"=path "D:/Phuc/Car_exel.xlsx") -> ()  [unwired: 12 in, 2 out]
                      }
                    }
                  }
                  frame #1 {
                    n241 = vi-ref "X4.vi"() -> (w265:refnum<vi>)
                    n242 = invoke class="VI" method="FP.Open"(reference=w265, "State"=T10."Maximized") -> (reference out=w263:refnum<vi>)  [unwired: 3 in, 4 out]
                    n243 = Close Reference(reference=w263) -> ()  [unwired: 1 in, 1 out]
                  }
                  frame #2 {
                    n244 = local read "GroupOpened"() -> (w266:bool)
                    n245 = case shown="True" w266 {
                      frame False {
                      }
                      frame True {
                        n246 = local read "GPHandle"() -> (w270:u64)
                        n247 = call <userlib>:"Acm_GpClose.vi"("pGpHandle"=w270) -> ("ReturnValue"=w268:u32)  [unwired: 1 in, 1 out]
                        n248 = Equal To 0?(x=w268) -> (x = 0?=w267:bool)
                        n249 = local write "GroupClosed"(w267) -> ()
                        n250 = case shown="True" w267 {
                          selector: w267 -> [_ w274]
                          frame False {
                          }
                          frame True {
                            n251 = Not(x=w274) -> (.not. x?=w273:bool)
                            n252 = local write "CFG_GpAxesInGroup"(u32 0 ("CFG_GpAxesInGroup")) -> ()
                            n253 = local write "GPHandle"(u32 0 ("GPHandle")) -> ()
                            n254 = local write "GroupOpened"(w273) -> ()
                            n255 = local write "DirectRelSuccess"(w273) -> ()
                            n256 = local write "GroupStopped"(w273) -> ()
                            n257 = local write "DirectAbsSuccess"(w273) -> ()
                          }
                        }
                        n258 = Not(x=w267) -> (.not. x?=w269:bool)
                        n259 = case shown="True" w269 {
                          tunnel: w268 -> [_ w278]
                          frame False {
                          }
                          frame True {
                            n260 = Number To Hexadecimal String(2:w278) -> (0:w276:string)  [unwired: 1 out]
                            n261 = Concatenate Strings("Group Close failed with Error Code:0x", w276) -> (w275:string)
                            n262 = One Button Dialog(message=w275) -> ()  [unwired: 2 out]
                          }
                        }
                      }
                    }
                  }
                  frame #3 {
                    n263 = local read "DevAxesCount"() -> (w279:u32)
                    n264 = for {
                      N: w279 -> [_]
                      i -> [w284]
                      n265 = local read "AxisHandle_Array"() -> (w285:u64[])
                      n266 = Index Array(array=w285, index=w284) -> (element=w283:u64)
                      n267 = call <userlib>:"Acm_AxClose.vi"("AxisHandle"=w283) -> ("ReturnValue"=w282:u32)  [unwired: 1 in, 1 out]
                      n268 = Equal To 0?(x=w282) -> (x = 0?=w281:bool)
                      n269 = Not(x=w281) -> (.not. x?=w280:bool)
                      n270 = local write "AxisOpened"(w280) -> ()
                    }
                  }
                  frame #4 {
                    n271 = local read "DeviceHandle"() -> (w288:u64)
                    n272 = call <userlib>:"Acm_DevClose.vi"("DeviceHandle"=w288) -> ("ReturnValue"=w287:u32)  [unwired: 1 in, 3 out]
                    n273 = Equal To 0?(x=w287) -> (x = 0?=w286:bool)
                    n274 = local write "CloseSuccess"(w286) -> ()
                    n275 = case shown="True" w286 {
                      tunnel: w286 -> [_ w291]
                      frame False {
                      }
                      frame True {
                        n276 = Not(x=w291) -> (.not. x?=w290:bool)
                        n277 = local write "GPHandle"(u32 0 ("GPHandle")) -> ()
                        n278 = local write "DevAxesCount"(u32 0 ("DevAxesCount")) -> ()
                        n279 = local write "DeviceHandle"(u32 0 ("DeviceHandle")) -> ()
                        n280 = local write "AxisOpened"(w290) -> ()
                        n281 = local write "DeviceOpened"(w290) -> ()
                        n282 = local write "ResetCounter"(w290) -> ()
                        n283 = local read "DevAxesCount"() -> (w294:u32)
                        n284 = Initialize Array(u32 0 ("元素"), w294) -> (w293:u32[])
                        n285 = local write "AxisHandle_Array"(w293) -> ()
                      }
                    }
                  }
                }
              }
              frame True {
              }
            }
          }
          frame #1 {
            n286 = call <vilib>:"Stop Timed Structure.vi"("name"=w297) -> ()  [unwired: 2 in, 9 out]
          }
        }
        "Exit Program" <- "Stop 2"
      }
      event "Set pos": Mouse Up {
        n287 = event-data() -> ()  [unwired: 2 out]
        n288 = Array Subset(array="Set cmd & actual pos", index=0, length=3) -> (w303:dbl[])
        n289 = Array Subset(array="Set cmd & actual pos", index=3, length=3) -> (w302:dbl[])
        n290 = Open MATLAB Session() -> (8:w310:refnum<k37>)  [unwired: 2 in, 1 out]
        n291 = node(w310, path "D:/New folder/postopulsemm.m" ("source file path"), dbl[] [], w303, w302) -> (w309:refnum<k37>, w299:dbl[])  [unwired: 4 in, 3 out]
        n292 = Close MATLAB Session(0:w309) -> ()  [unwired: 1 in, 1 out]
        n293 = local read "DevAxesCount"() -> (w298:u32)
        n294 = for {
          N: w298 -> [_]
          tunnel: w299 -> [w313]
          i -> [w314]
          n295 = local read "AxisHandle_Array"() -> (w316:u64[])
          n296 = Index Array(array=w313, index=w314) -> (element=w312:dbl)
          n297 = expression code="x*125/16"(w312) -> (w311:dbl)
          n298 = Index Array(array=w316, index=w314) -> (element=w315:u64)
          n299 = call <userlib>:"Acm_AxSetActualPosition.vi"("Position"=w311, "AxisHandle"=w315) -> ()  [unwired: 1 in, 3 out]
          n300 = call <userlib>:"Acm_AxSetCmdPosition.vi"("Position"=w312, "AxisHandle"=w315) -> ()  [unwired: 1 in, 3 out]
        }
      }
    }
  }
  n301 = node-c288(w27) -> (w29:T11)  [unwired: 2 in, 3 out]
  n302 = timed-loop {
    timing: w29 -> [_]
    timing-out: [_] -> w28
    stop <- _ stop-if-true
    n303 = node-c288() -> ()  [unwired: 2 out]
    n304 = local read "DeviceOpened"() -> (w319:bool)
    n305 = local read "AxisOpened"() -> (w318:bool)
    n306 = And(x=w319, y=w318) -> (x .and. y?=w317:bool)
    n307 = case shown="True" w317 {
      frame False {
      }
      frame True {
        n308 = local read "GroupOpened"() -> (w320:bool)
        n309 = case shown="True" w320 {
          frame False {
          }
          frame True {
            n310 = local read "GPHandle"() -> (w325:u64)
            n311 = local read "DeviceHandle"() -> (w324:u64)
            n312 = call <userlib>:"CFG_GpAxesInGroup.vi"("Handle"=w325) -> ("CFG_GpAxesInGroup"=→"CFG_GpAxesInGroup":u32)  [unwired: 1 in, 13 out]
            n313 = call <userlib>:"Acm_GpGetState.vi"("GpHandle"=w325) -> ("ReturnValue"=w329:u32, "pState"=w323:u16)  [unwired: 1 in, 3 out]
            n314 = Equal To 0?(x=w329) -> (x = 0?=w328:bool)
            n315 = Equal?(x=w323, y=u16 6) -> (x = y?=→"Ax = y?":bool)
            n316 = for {
              N: 2 -> [_]
              tunnel: w324 -> [w333]
              tunnel: w325 -> [w332]
              i -> [w334]
              n317 = case shown="0, Default" w334 {
                tunnel: [w340 w342] -> w331
                tunnel: w333 -> [w339 _]
                tunnel: w332 -> [_ w341]
                frame 0, Default {
                  n318 = call <userlib>:"Acm_GetLastError.vi"("ObjectHandle"=w339) -> ("ReturnValue"=w340:u32)  [unwired: 1 in, 2 out]
                }
                frame 1 {
                  n319 = call <userlib>:"Acm_GetLastError.vi"("ObjectHandle"=w341) -> ("ReturnValue"=w342:u32)  [unwired: 1 in, 2 out]
                }
              }
              n320 = Not Equal To 0?(x=w331) -> (x != 0?=w330:bool)
              n321 = case shown="True" w330 {
                selector: w330 -> [_ w335]
                tunnel: w331 -> [_ w336]
                frame False {
                }
                frame True {
                  n322 = call <userlib>:"Acm_GetErrorMessage.vi"("nMaxError"=50) -> ("ErrorMsg"=→"Error Msg":string)  [unwired: 1 in, 4 out]
                  "Error Code:" <- w336
                  "Error" <- w335
                }
              }
            }
            n323 = case shown="True" w328 {
              tunnel: w323 -> [_ w343]
              frame False {
              }
              frame True {
                n324 = case shown="0, Default" w343 {
                  frame 0, Default {
                    "Group State:" <- "Group is disabled." ("Axis State:")
                  }
                  frame 1 {
                    n325 = local write "Group State:"("Group is ready." ("Axis State:")) -> ()
                  }
                  frame 2 {
                    n326 = local write "Group State:"("Group is stopping." ("Axis State:")) -> ()
                  }
                  frame 3 {
                    n327 = local write "Group State:"("Group is Error_Stopped." ("Axis State:")) -> ()
                  }
                  frame 4 {
                    n328 = local write "Group State:"("Group is executing interpolation motion." ("Axis State:")) -> ()
                  }
                  frame 5 {
                    n329 = local write "Group State:"("Axis(Axes) in Group is(are) executing single axis motion." ("Axis State:")) -> ()
                  }
                  frame 6 {
                    n330 = local write "Group State:"("Group is executing continuous interpolation motion(Path)." ("Axis State:")) -> ()
                  }
                }
              }
            }
          }
        }
      }
    }
    n331 = node-c288() -> ()  [unwired: 2 out]
  }
  n332 = node-c288(w28) -> ()  [unwired: 1 out]
  n333 = TCP Open Connection(address="Address", remote port or service name="Port") -> (connection ID=w12:refnum<k5>, error out=w11:errorcluster)  [unwired: 3 in]
  n334 = call <vilib>:"Connect.vi"("trust any server (F)"="trust any server (F)", "security policy"=T5 {"message mode"=enum."Sign", "security"=enum."Basic256"}, "server endpoint URL"="Server endpoint URL") -> ("OPC UA client refnum out"=w7:T14)  [unwired: 6 in, 2 out]
  n335 = while {
    shift-right: [w380] -> w23
    shift-left: w21 -> [w387]
    shift-right: [w381] -> w24
    shift-left: w22 -> [w386]
    tunnel: w15 -> [w379]
    tunnel: [w360] -> w4
    tunnel: [w357] -> w3
    tunnel: [w356] -> w2
    tunnel: [w353] -> w1
    stop <- w378 stop-if-true
    n336 = call <extravilib>:"Read.vi"("channel"=w379) -> ("element"=w378:bool)  [unwired: 1 in, 1 out]
    n337 = TCP Write(connection ID=w387, data in="kakaka", error in (no error)=w386) -> (connection ID out=w385:refnum<k5>, error out=w383:errorcluster)  [unwired: 1 in, 1 out]
    n338 = TCP Read(connection ID=w385, bytes to read="bytes to read 2", error in (no error)=w383) -> (connection ID out=w380:refnum<k5>, data out=w361:string, error out=w381:errorcluster)  [unwired: 2 in]
    "data out 2" <- w361
    n339 = String Subset(string=w361, offset (0)=0, length (rest)=8 ("length (rest)")) -> (substring=w373:string)
    n340 = String Subset(string=w361, offset (0)=8, length (rest)=8 ("length (rest)")) -> (substring=w368:string)
    n341 = String Subset(string=w361, offset (0)=24, length (rest)=8 ("length (rest)")) -> (substring=w362:string)
    n342 = String Subset(string=w361, offset (0)=16, length (rest)=8 ("length (rest)")) -> (substring=w364:string)
    n343 = Scan Value(string=w373, format string="%f") -> ()  [unwired: 1 in, 2 out]
    n344 = Scan Value(string=w368, format string="%f") -> ()  [unwired: 1 in, 2 out]
    n345 = Scan Value(string=w362, format string="%f") -> (value=w358:dbl)  [unwired: 1 in, 1 out]
    n346 = Scan Value(string=w364, format string="%f") -> (value=w354:dbl)  [unwired: 1 in, 1 out]
    n347 = call <extravilib>:"Write.vi"("element"=w358) -> ("channel"=w357:T15)  [unwired: 1 out]
    n348 = call <extravilib>:"Write.vi"("element"=w354) -> ("channel"=w353:T15)  [unwired: 1 out]
    n349 = call <extravilib>:"Write.vi"("element"=0.0) -> ("channel"=w360:T15)  [unwired: 1 out]
    n350 = call <extravilib>:"Write.vi"("element"=0.0) -> ("channel"=w356:T15)  [unwired: 1 out]
  }
  n351 = TCP Close Connection(connection ID=w23, error in (no error)=w24) -> ()  [unwired: 1 in, 2 out]
  n352 = while {
    tunnel: [w430] -> w15
    tunnel: [w425] -> w16
    tunnel: w4 -> [w406]
    tunnel: w3 -> [w405]
    tunnel: w2 -> [w403]
    tunnel: w1 -> [w401]
    stop <- "Stop 3" stop-if-true
    n353 = call <extravilib>:"Read.vi"("channel"=w405) -> ("element"=w404:dbl)  [unwired: 1 in, 1 out]
    n354 = call <extravilib>:"Read.vi"("channel"=w401) -> ("element"=w400:dbl)  [unwired: 1 in, 1 out]
    n355 = call <extravilib>:"Read.vi"("channel"=w403) -> ("element"=w402:dbl)  [unwired: 1 in, 1 out]
    n356 = call <extravilib>:"Read.vi"("channel"=w406) -> ("element"=w394:dbl)  [unwired: 1 in, 1 out]
    "angle Y" <- w394
    n357 = expression code="x-0.111111"(w404) -> (w410:dbl)
    n358 = expression code="x-0.111111"(w400) -> (w390:dbl)
    "vx" <- w390
    "velx" <- w390
    n359 = local read "GroupOpened"() -> (w426:bool)
    n360 = local read "GroupOpened"() -> (w427:bool)
    n361 = local read "GPHandle"() -> (w428:u64)
    n362 = In Range and Coerce(upper limit=400.0, x=w410, lower limit=-400.0) -> (coerced(x)=w391:dbl)  [unwired: 1 out]
    "x" <- w391
    "x" <- w391
    n363 = case shown="True" w426 {
      frame False {
      }
      frame True {
        n364 = local read "pRemainCount"() -> (w433:u32)
        n365 = local read "Ax = y?"() -> (w435:bool)
        n366 = Not(x=w435) -> (.not. x?=w437:bool)
        n367 = local read "GPHandle"() -> (w432:u64)
        n368 = Greater?(x=w433, y=u32 0) -> (0:w436:bool)
        n369 = And(x=w436, y=w437) -> (x .and. y?=w431:bool)
        n370 = case shown="True" w431 {
          tunnel: w432 -> [_ w438]
          frame False {
          }
          frame True {
            n371 = call <userlib>:"Acm_GpMovePath.vi"("PathHandle"=u64 0, "GpHandle"=w438) -> ()  [unwired: 1 in, 4 out]
          }
        }
      }
    }
    n372 = case shown="True" w427 {
      tunnel: w428 -> [_ w443]
      frame False {
      }
      frame True {
        n373 = call <userlib>:"Acm_GpGetPathStatus.vi"("GpHandle"=w443) -> ("GpHandle"=w444:u64, "pCurIndex"=→"pCurIndex":u32, "pCurCmdFunc"=→"pCurCmdFunc":u32, "pRemainCount"=w440:u32, "pFreeSpaceCount"=→"pFreeSpaceCount":u32)  [unwired: 20 in, 2 out]
        "pRemainCount" <- w440
        n374 = Greater?(x=w440, y="y") -> (0:w442:bool)
        n375 = case shown="False" w442 {
          tunnel: w444 -> [w448 _]
          tunnel: w440 -> [_ _]
          frame False {
            n376 = stacked-sequence {
              tunnel: w448 -> [_ w464]
              frame #0 {
                n377 = local read "GPHandle"() -> (w450:u64)
                n378 = call <userlib>:"CFG_GpBldTime.vi"("CFG_GpBldTime"="CFG_GpBldTime", "Handle"=w450) -> ("Handle 2"=w451:u64)  [unwired: 1 in, 2 out]
                n379 = call <userlib>:"CFG_GpSFEnable.vi"("CFG_GpSFEnable"="CFG_GpSFEnable", "Handle"=w451) -> ()  [unwired: 1 in, 3 out]
              }
              frame #1 {
                w462 = u16 1 items=["Enable blending", "Disable bleding"] ("MoveMode")
                w463 = u16 84 items=["EndPath"=0, "Abs2DLine"=1, "Rel2DLine"=2, "Abs2DArcCW"=3, "Abs2DArcCCW"=4, "Rel2DArcCW"=5, "Rel2DArcCCW"=6, "Abs3DLine"=7, "Rel3DLine"=8, "Abs4DLine"=9, "Rel4DLine"=10, "Abs2DDirect"=11, "Rel2DDirect"=12, "Abs3DDirect"=13, "Rel3DDirect"=14, "Abs4DDirect"=15, "Rel4DDirect"=16, "Abs5DDirect"=17, "Rel5DDirect"=18, "Abs6DDirect"=19, "Rel6DDirect"=20, "Abs3DArcCW"=21, "Rel3DArcCW"=22, "Abs3DArcCCW"=23, "Rel3DArcCCW"=24, "Abs3DHelixCW"=25, "Rel3DHelixCW"=26, "Abs3DHelixCCW"=27, "Rel3DHelixCCW"=28, "GPDELAY"=29, "Abs4DSpiralCW"=30, "Rel4DSpiralCW"=31, "Abs4DSpiralCCW"=32, "Rel4DSpiralCCW"=33, "Abs5DSpiralCW"=34, "Rel5DSpiralCW"=35, "Abs5DSpiralCCW"=36, "Rel5DSpiralCCW"=37, "Abs6DSpiralCW"=38, "Rel6DSpiralCW"=39, "Abs6DSpiralCCW"=40, "Rel6DSpiralCCW"=41, "Abs7DSpiralCW"=42, "Rel7DSpiralCW"=43, "Abs7DSpiralCCW"=44, "Rel7DSpiralCCW"=45, "Abs8DSpiralCW"=46, "Rel8DSpiralCW"=47, "Abs8DSpiralCCW"=48, "Rel8DSpiralCCW"=49, "Abs8DDirect"=84, "Rel8DDirect"=85] ("MoveCmd")
                n380 = local read "Operate Axes"() -> (w460:T3)
                n381 = local read "DevAxesCount"() -> (w457:u32)
                n382 = Cluster To Array(cluster=w460) -> (array=w459:bool[])
                n383 = Boolean Array To Number(Boolean array=w459) -> (number=w458:u32)
                n384 = for {
                  N: w457 -> [_]
                  tunnel: w458 -> [w469]
                  shift-right: [w465] -> w455
                  shift-left: u32 0 -> [w466]
                  i -> [w467]
                  n385 = formula code="uInt32 y;\n\ny=(x>>i) & 0x01;"("x"=w469, "i"=w467) -> ("y"=w468:u32)
                  n386 = case shown="0, Default" w468 {
                    tunnel: w466 -> [w471 w474]
                    tunnel: [w470 w473] -> w465
                    frame 0, Default {
                      n387 = Add(x=w471, y=u32 0) -> (x+y=w470:u32)
                    }
                    frame 1 {
                      n388 = Increment(x=w474) -> (x+1=w473:u32)
                    }
                  }
                }
                n389 = local read "Endpoint_Highqq"() -> (w454:dbl)
                n390 = local read "Endpoint_l"() -> (w453:dbl[])
                n391 = call <userlib>:"Acm_GpAddPath.vi"("GPHandle"=w464, "MoveCmd"=w463, "MoveMode"=w462, "FH"=w454, "FL"=0.0, "EndPoint_DataArray"=w453, "ArrayElements"=w455) -> ()  [unwired: 18 in, 3 out]
              }
            }
          }
          frame True {
          }
        }
      }
    }
    n392 = Initialize Array(0.0 ("element"), 4 ("dimension size")) -> (w422:dbl[])
    n393 = Build Array (concatenate)(w390, w422, w402) -> (w399:dbl[])
    "appended array 2" <- w399
    n394 = Build Array(w391, 0.0 ("element"), 100.0 ("element"), 0.0 ("element"), w394, 0.0 ("element")) -> (w392:dbl[])
    "appended array" <- w392
    n395 = Open MATLAB Session() -> (8:w421:refnum<k37>)  [unwired: 2 in, 1 out]
    n396 = Build Array(w391, w390) -> (w398:dbl[])
    n397 = node(w421, "source file path", T16 {"Endpoint_lfull"=[], "Endpoint_l"=[], "Endpoint_Highqq"=0.0}, w392, w399) -> (w420:refnum<k37>, w417:T16)  [unwired: 4 in, 3 out]
    n398 = Close MATLAB Session(0:w420) -> ()  [unwired: 1 in, 1 out]
    n399 = Unbundle By Name(w417) -> ("Endpoint_lfull"=→"Endpoint_lfull 2":dbl[][], "Endpoint_l"=→"Endpoint_l":dbl[], "Endpoint_Highqq"=w414:dbl)
    n400 = expression code="x*100"(w414) -> (w413:dbl)
    n401 = Multiply(x=w413, y="y 2") -> (x*y=w389:dbl)
    n402 = In Range and Coerce(upper limit=64000.0, x=w389, lower limit=10000.0) -> (coerced(x)=→"Endpoint_Highqq" →"highqq":dbl)  [unwired: 1 out]
    n403 = case shown="True" "Stop 3" {
      frame False {
      }
      frame True {
        n404 = local read "GPHandle"() -> (w475:u64)
        n405 = call <userlib>:"Acm_GpStopEmg.vi"("GpHandle"=w475) -> ()  [unwired: 1 in, 3 out]
      }
    }
    n406 = call <extravilib>:"Write.vi"("element"=w398) -> ("channel"=w425:T17)  [unwired: 1 out]
    n407 = call <extravilib>:"Write.vi"("element"="Stop 3") -> ("channel"=w430:T18)  [unwired: 1 out]
  }
  n408 = while {
    tunnel: w16 -> [w491]
    shift-right: [w479] -> _
    shift-left: dbl[][] [] -> [w482]
    tunnel: w15 -> [w489]
    tunnel: [w487] -> w5
    stop <- w488 stop-if-true
    n409 = call <extravilib>:"Read.vi"("channel"=w491) -> ("element"=w490:dbl[])  [unwired: 1 in, 1 out]
    n410 = call <extravilib>:"Read.vi"("channel"=w489) -> ("element"=w488:bool)  [unwired: 1 in, 1 out]
    n411 = local read "Cable length Array"() -> (w476:dbl[])
    n412 = local read "Tensile force array"() -> (w481:dbl[])
    n413 = local read "Tilt sensor array"() -> (w480:dbl[])
    n414 = local read "Gyro acc & vel"() -> (w477:dbl[])
    n415 = Wait Until Next ms Multiple(millisecond multiple=u32 100) -> ()  [unwired: 1 out]
    n416 = case shown="True" "Enable write" {
      tunnel: w490 -> [_ w512]
      tunnel: [w507 w516] -> w485
      tunnel: w482 -> [w507 w515]
      tunnel: w476 -> [_ w514]
      tunnel: w481 -> [_ w513]
      tunnel: w480 -> [_ w511]
      tunnel: w477 -> [_ w510]
      frame False {
      }
      frame True {
        n417 = Tick Count (ms)() -> (millisecond timer value=w509:u32)
        n418 = To Double Precision Float(number=w509) -> (double precision float=w508:dbl)
        n419 = Build Array (concatenate)(w508, w511, w512, w514, w513, w510) -> (w517:dbl[])
        n420 = Build Array (concatenate)(w515, w517) -> (w516:dbl[][])
      }
    }
    n421 = case shown="True" "Clear report" {
      tunnel: [w504 dbl[][] []] -> w479
      tunnel: w485 -> [w504 _]
      frame False {
      }
      frame True {
        n422 = local read "Exel report"() -> (w506:refnum<class "NI_report.lvclass">)
        n423 = call-dynamic "Clear Report.vi"("report in"=w506) -> ()  [unwired: 13 in, 2 out]
      }
    }
    n424 = case shown="True" "Write to report" {
      tunnel: w479 -> [_ w500]
      frame False {
      }
      frame True {
        n425 = local read "Exel report"() -> (w501:refnum<class "NI_report.lvclass">)
        n426 = Current VI's Path() -> (path=w499:path)
        n427 = Concatenate Strings("String", ".csv" ("string")) -> (w494:string)
        n428 = Strip Path(path=w499) -> (stripped path=w497:path)  [unwired: 1 out]
        n429 = Build Path(base path=w497, name or relative path=w494) -> (appended path=w498:path)
        n430 = call-poly <vilib>:"Append Table to Report.vi"("report in"=w501, "MS Office parameters"=T19 {"position (excel)"={"row"=1, "column"=0}, "name (excel)"="", "bookmark (word)"=""}, "numerical data"=w500, "format string (%.3f)"="%.3f") -> ()  [unwired: 8 in, 4 out]
        n431 = call-poly <vilib>:"Write Delimited Spreadsheet.vi"("file path (dialog if empty)"=w498, "format (%.3f)"="%.3f", "2D data"=w500, "delimiter (\\t)"="," ("delimiter (\\t)")) -> ()  [unwired: 10 in, 2 out]
      }
    }
    n432 = call <extravilib>:"Write.vi"("element"=w488) -> ("channel"=w487:T18)  [unwired: 1 out]
  }
  n433 = while {
    tunnel: w12 -> [w574]
    tunnel: w11 -> [w573]
    tunnel: [w572] -> w10
    tunnel: [w571] -> w9
    tunnel: w5 -> [w570]
    stop <- w553 stop-if-true
    w535 = "%.3f" ("format string")
    w518 = "%.3f" ("format string")
    n434 = call <extravilib>:"Read.vi"("channel"=w570) -> ("element"=w553:bool)  [unwired: 1 in, 1 out]
    n435 = TCP Read(connection ID=w574, bytes to read="bytes to read", error in (no error)=w573) -> (connection ID out=w572:refnum<k5>, data out=w536:string, error out=w571:errorcluster)  [unwired: 2 in]
    "data out" <- w536
    n436 = String Subset(string=w536, offset (0)=1, length (rest)=7 ("length (rest)")) -> (substring=w554:string)
    n437 = String Subset(string=w536, offset (0)=9, length (rest)=7 ("length (rest)")) -> (substring=w569:string)
    "Pitch" <- w569
    n438 = String Subset(string=w536, offset (0)=17, length (rest)=7 ("length (rest)")) -> (substring=w568:string)
    n439 = String Subset(string=w536, offset (0)=25, length (rest)=7 ("length (rest)")) -> (substring=w534:string)
    "LinAcc X" <- w534
    n440 = String Subset(string=w536, offset (0)=33, length (rest)=7 ("length (rest)")) -> (substring=w533:string)
    "LinAcc Y" <- w533
    n441 = String Subset(string=w536, offset (0)=41, length (rest)=7 ("length (rest)")) -> (substring=w532:string)
    "LinAcc Z" <- w532
    n442 = String Subset(string=w536, offset (0)=56, length (rest)=8 ("length (rest)")) -> (substring=w538:string)
    n443 = String Subset(string=w536, offset (0)=48, length (rest)=8 ("length (rest)")) -> (substring=w539:string)
    n444 = String Subset(string=w536, offset (0)=64, length (rest)=8 ("length (rest)")) -> (substring=w537:string)
    n445 = Scan Value(string=w554, format string=w518) -> (value=w555:dbl)  [unwired: 1 in, 1 out]
    n446 = Scan Value(string=w569, format string=w518) -> (value=w563:dbl)  [unwired: 1 in, 1 out]
    n447 = Scan Value(string=w568, format string=w518) -> (value=w566:dbl)  [unwired: 1 in, 1 out]
    n448 = Add(x=w555, y=179.7) -> (x+y=w559:dbl)
    n449 = Subtract(x=180.25, y=w555) -> (x-y=w557:dbl)
    n450 = Scan Value(string=w534, format string=w535) -> (value=w529:dbl)  [unwired: 1 in, 1 out]
    n451 = Scan Value(string=w533, format string=w535) -> (value=w530:dbl)  [unwired: 1 in, 1 out]
    n452 = Scan Value(string=w532, format string=w535) -> (value=w531:dbl)  [unwired: 1 in, 1 out]
    n453 = Scan Value(string=w538, format string=w535) -> (value=w523:dbl)  [unwired: 1 in, 1 out]
    n454 = Scan Value(string=w539, format string=w535) -> (value=w522:dbl)  [unwired: 1 in, 1 out]
    n455 = Scan Value(string=w537, format string=w535) -> (value=w519:dbl)  [unwired: 1 in, 1 out]
    n456 = expression code="x+0.025"(w519) -> (w520:dbl)
    n457 = expression code="x-0.02"(w529) -> (w526:dbl)
    n458 = expression code="x-0.02"(w530) -> (w527:dbl)
    n459 = expression code="x-0.01"(w531) -> (w528:dbl)
    n460 = expression code="x+1.3"(w523) -> (w524:dbl)
    n461 = expression code="x+0.1"(w522) -> (w521:dbl)
    n462 = Negate(x=w559) -> (-x=w552:dbl)
    n463 = Greater?(x=w555, y=0.0) -> (0:w561:bool)
    n464 = expression code="(x+73.3)*3"(w566) -> (w565:dbl)
    n465 = Select(t=w557, s=w561, f=w552) -> (s? t:f=w556:dbl)
    n466 = Build Array(w526, w527, w528, w524, w521, w520) -> (→"Gyro acc & vel":dbl[])
    n467 = Negate(x=w556) -> (-x=w549:dbl)
    n468 = Subtract(x=w563, y=1.08) -> (x-y=w548:dbl)
    n469 = Build Array(w549, w548) -> (w547:dbl[])
    n470 = Build Array(w549, w548, w565) -> (→"Tilt sensor array":dbl[])
    n471 = Format Into String(format string="%.2f", w549) -> (resulting string=→"Roll":string)  [unwired: 2 in, 1 out]
    n472 = Array To Cluster(array=w547) -> (cluster=→"Roll & Pitch":cluster{"[0]":dbl, "[1]":dbl})
  }
  n473 = while {
    tunnel: w7 -> [w598]
    tunnel: [w597] -> w6
    tunnel: w5 -> [w596]
    stop <- w595 stop-if-true
    n474 = call <extravilib>:"Read.vi"("channel"=w596) -> ("element"=w595:bool)  [unwired: 1 in, 1 out]
    n475 = Build Array("NodeID 1", "NodeID 2", "NodeID 3", "NodeID 4", "NodeID 5", "NodeID 6", "NodeID 7", "NodeID 8") -> (w612:string[])
    n476 = call-poly <vilib>:"Multiple Read.vi"("node IDs"=w612, "OPC UA client refnum in"=w598) -> ("results"=w617:T22, "OPC UA client refnum out"=w597:T14)  [unwired: 6 in, 2 out]
    n477 = Index Array(array=w617) -> (element #1=w611:T23, element #2=w594:T23, element #3=w593:T23, element #4=w592:T23, element #5=w591:T23, element #6=w590:T23, element #7=w589:T23, element #8=w588:T23)  [unwired: 8 in]
    n478 = Unbundle By Name(w611) -> ("value"=w610:sgl)  [unwired: 1 out]
    n479 = Unbundle By Name(w594) -> ("value"=w609:sgl)  [unwired: 1 out]
    n480 = Unbundle By Name(w593) -> ("value"=w608:sgl)  [unwired: 1 out]
    n481 = Unbundle By Name(w592) -> ("value"=w607:sgl)  [unwired: 1 out]
    n482 = Unbundle By Name(w591) -> ("value"=w602:sgl)  [unwired: 1 out]
    n483 = Unbundle By Name(w590) -> ("value"=w601:sgl)  [unwired: 1 out]
    n484 = Unbundle By Name(w589) -> ("value"=w600:sgl)  [unwired: 1 out]
    n485 = Unbundle By Name(w588) -> ("value"=w599:sgl)  [unwired: 1 out]
    n486 = Build Array(w610, w609, w608, w607, w602, w601, w600, w599) -> (w619:sgl[])
    n487 = expression code="x*9.8"(w619) -> (w620:sgl[])
    "Tensile force array" <- w620
    n488 = Array To Cluster(array=w620) -> (cluster=→"Measured tensile force (N)":T2)
  }
  n489 = call <vilib>:"Disconnect.vi"("OPC UA client refnum in"=w6) -> ()  [unwired: 10 in, 1 out]
  n490 = TCP Close Connection(connection ID=w10, error in (no error)=w9) -> ()  [unwired: 1 in, 2 out]
